vi "#32_MAV_MSG_LOCAL_POSITION_NED_DECODE.vi"(11 "mavlink_payload":u8[](array[numeric])) -> (3 "LOCAL_POSITION_NED":T1)   [LabVIEW 2023]
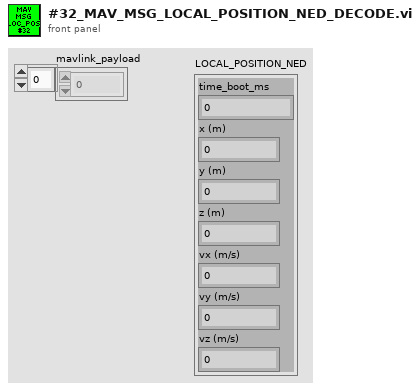
[diagram p1: front panel]
types:
  T1 = cluster{"time_boot_ms":u32, "x (m)":sgl, "y (m)":sgl, "z (m)":sgl, "vx (m/s)":sgl, "vy (m/s)":sgl, "vz (m/s)":sgl}
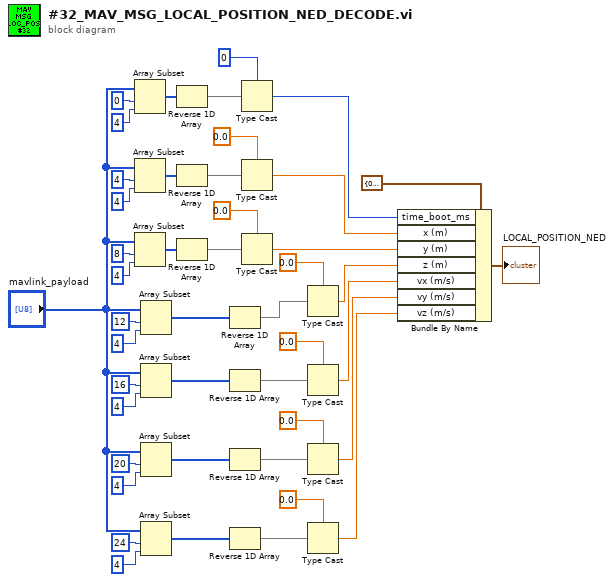
[diagram p0: block diagram]
diagram:
  n1 = Array Subset(array="mavlink_payload", index=0, length=4) -> (w45:u8[])
  n2 = Array Subset(array="mavlink_payload", index=4, length=4) -> (w37:u8[])
  n3 = Array Subset(array="mavlink_payload", index=8, length=4) -> (w31:u8[])
  n4 = Array Subset(array="mavlink_payload", index=12, length=4) -> (w26:u8[])
  n5 = Array Subset(array="mavlink_payload", index=16, length=4) -> (w19:u8[])
  n6 = Array Subset(array="mavlink_payload", index=20, length=4) -> (w13:u8[])
  n7 = Array Subset(array="mavlink_payload", index=24, length=4) -> (w7:u8[])
  n8 = Reverse 1D Array(array=w45) -> (reversed array=w44:u8[])
  n9 = Reverse 1D Array(array=w37) -> (reversed array=w36:u8[])
  n10 = Reverse 1D Array(array=w31) -> (reversed array=w30:u8[])
  n11 = Reverse 1D Array(array=w26) -> (reversed array=w25:u8[])
  n12 = Reverse 1D Array(array=w19) -> (reversed array=w18:u8[])
  n13 = Reverse 1D Array(array=w13) -> (reversed array=w12:u8[])
  n14 = Reverse 1D Array(array=w7) -> (reversed array=w6:u8[])
  n15 = Type Cast(type=u32 0 ("index"), x=w44) -> (*(type *) &x=w38:u32)
  n16 = Type Cast(type=sgl 0.0 ("index"), x=w36) -> (*(type *) &x=w32:sgl)
  n17 = Type Cast(type=sgl 0.0 ("index"), x=w30) -> (*(type *) &x=w21:sgl)
  n18 = Type Cast(type=sgl 0.0 ("index"), x=w25) -> (*(type *) &x=w20:sgl)
  n19 = Type Cast(type=sgl 0.0 ("index"), x=w18) -> (*(type *) &x=w14:sgl)
  n20 = Type Cast(type=sgl 0.0 ("index"), x=w12) -> (*(type *) &x=w8:sgl)
  n21 = Type Cast(type=sgl 0.0 ("index"), x=w6) -> (*(type *) &x=w2:sgl)
  n22 = Bundle By Name(cluster=T1 {"time_boot_ms"=0, "x (m)"=0.0, "y (m)"=0.0, "z (m)"=0.0, "vx (m/s)"=0.0, "vy (m/s)"=0.0, "vz (m/s)"=0.0} ("LOCAL_POSITION_NED"), "time_boot_ms"=w38, "x (m)"=w32, "y (m)"=w21, "z (m)"=w20, "vx (m/s)"=w14, "vy (m/s)"=w8, "vz (m/s)"=w2) -> (→"LOCAL_POSITION_NED":T1)
